vi "GetModules_Boolean.vi"(9 "Boolean in":refnum<class "Boolean.lvclass">) -> (3 "Boolean out":refnum<class "Boolean.lvclass">, 4 "modules":T1[](array[typedef]))   [LabVIEW 2014, in "Raspberry Pi Compatible Compiler for LabVIEW.lvlib" / "PythonConverter_GUI.lvclass"]
uses:
  PythonConverter_GUI.lvclass
  VI Interpreter/Classes/Boolean/Boolean.lvclass
  TypeDefs/PythonModuleTD.ctl
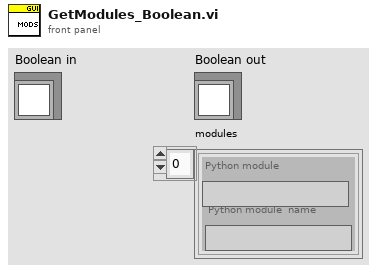
[diagram p1: front panel]
types:
  T1 = typedef "Raspberry Pi Compatible Compiler for LabVIEW.lvlib/PythonConverter_GUI.lvclass/PythonModuleTD.ctl" = cluster{"Python module":string, "Python module  name":string}
  T2 = cluster{"Python module  name":string, "Python module":string}[]
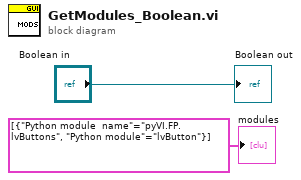
[diagram p0: block diagram]
diagram:
  "Boolean out" <- "Boolean in"
  "modules" <- T2 [{"Python module  name"="pyVI.FP.lvButtons", "Python module"="lvButton"}] ("modules")
